vi "ToString.vi"(8 "error in (no error)":errorcluster, 11 "ErrorMessageContains in":refnum<class "ErrorMessageContains.lvclass">) -> (0 "error out":errorcluster, 2 "String":string, 3 "ErrorMessageContains out":refnum<class "ErrorMessageContains.lvclass">)   [LabVIEW 2017, in "Transparent Assertions.lvlib" / "Constraints.lvlib" / "ErrorMessageContains.lvclass"]
doc: "Returns a string representation of the object."
uses:
  ErrorMessageContains.lvclass
  ErrorMessageContains.lvclass/ErrorMessageContains.ctl
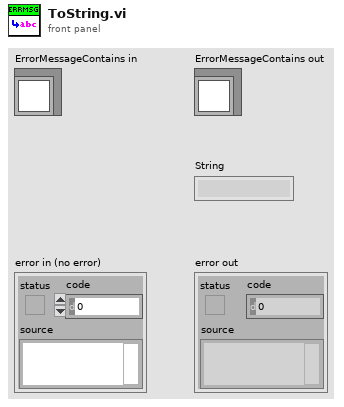
[diagram p1: front panel]
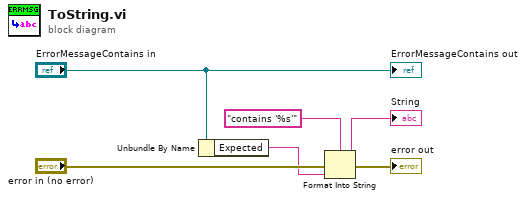
[diagram p0: block diagram]
diagram:
  n1 = Unbundle By Name("ErrorMessageContains in") -> ("Expected"=w1:string)
  n2 = Format Into String(format string="contains '%s'" ("String"), error in="error in (no error)", w1) -> (resulting string=→"String":string, error out=→"error out":errorcluster)  [unwired: 1 in]
  "ErrorMessageContains out" <- "ErrorMessageContains in"
